vi "Project Save for Previous.vi"(7 "LabVIEW Previous Version":T1=enum."2015", 8 "Error In":errorcluster) -> (0 "Error Out":errorcluster, 3 "Destination":path)   [LabVIEW 2017, in "Scripts.lvlib"]
doc: "Saves a project to a previous version of LabVIEW. The output is saved to \"<project root>\\target\\<Target Version>\", where \"<project root>\" is the folder that contains the LabVIEW project file (.lvproj) and \"<Target Version>\" is the previous version of LabVIEW, such as \"15.0\" for LabVIEW 2015."
uses:
  Scripts.lvlib
  Controls/LabVIEW Versions.ctl
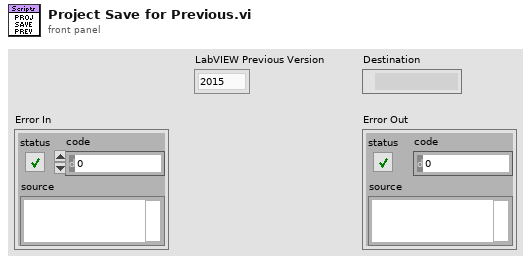
[diagram p1: front panel]
types:
  T1 = typedef "Scripts.lvlib/LabVIEW Versions.ctl" = enum16{"2009", "2010", "2011", "2012", "2013", "2014", "2015", "2016", "2017", "2018"}
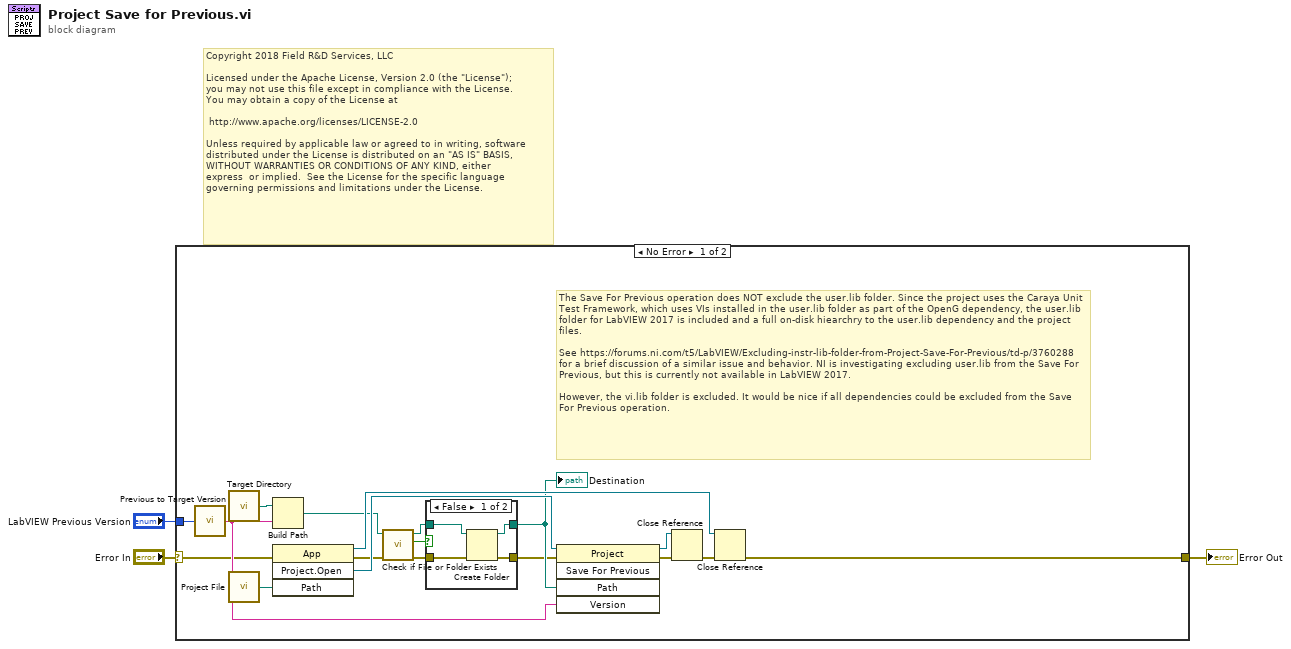
[diagram p0: block diagram]
diagram:
  # "Copyright 2018 Field R&D Services, LLC\n\nLicensed under the Apache License, Version 2.0 (the \"License\");\nyou may not use this file except in compliance with the License.\nYou may obtain a copy of the License at\n\n\thttp://www.apache.org/licenses/LICENSE-2.0\n\nUnless required by applicable law or agreed to in writing, software\ndistributed under the License is distributed on an \"AS IS\" BASIS,\nWITHOUT WARRANTIES OR CONDITIONS OF ANY KIND, either \nexpress  or implied.  See the License for the specific language \ngoverning permissions and limitations under the License."
  n1 = case shown="No Error" "Error In" {
    selector: "Error In" -> [w4 w28]
    tunnel: [w16 w28] -> w3
    tunnel: "LabVIEW Previous Version" -> [w9 _]
    frame No Error {
      # "The Save For Previous operation does NOT exclude the user.lib folder. Since the project uses the Caraya Unit Test Framework, which uses VIs installed in the user.lib folder as part of the OpenG dependency, the user.lib folder for LabVIEW 2017 is included and a full on-disk hiearchry to the user.lib dependency and the project files.\n\nSee https://forums.ni.com/t5/LabVIEW/Excluding-instr-lib-folder-from-Project-Save-For-Previous/td-p/3760288 for a brief discussion of a similar issue and behavior. NI is investigating excluding user.lib from the Save For Previous, but this is currently not available in LabVIEW 2017.\n\nHowever, the vi.lib folder is excluded. It would be nice if all dependencies could be excluded from the Save For Previous operation."
      n2 = call "Previous to Target Version.vi"("Previous Version"=w9) -> ("Target Version"=w7:string)
      n3 = call "Target Directory.vi"() -> ("Target Directory"=w5:path)
      n4 = call "Project File.vi"() -> ("Project File"=w6:path)
      n5 = Build Path(base path=w5, name or relative path=w7) -> (appended path=w8:path)
      n6 = invoke class="App" method="Project.Open"(error in=w4, "Path"=w6) -> (reference out=w18:refnum<vi>, error out=w15:errorcluster, "Project:Open"=w21:refnum<vi>)  [unwired: 2 in, 1 out]
      n7 = call <vilib>:"Check if File or Folder Exists.vi"("error in (no error)"=w15, "path"=w8) -> ("error out"=w11:errorcluster, "file or folder exists?"=w14:bool, "dup path"=w13:path)  [unwired: 7 in]
      n8 = case shown="False" w14 {
        tunnel: w13 -> [w25 w27]
        tunnel: [w22 w27] -> w12
        tunnel: w11 -> [w24 w26]
        tunnel: [w23 w26] -> w10
        frame False {
          n9 = Create Folder(path (use dialog)=w25, error in=w24) -> (created path=w22:path, error out=w23:errorcluster)  [unwired: 1 in, 1 out]
        }
        frame True {
        }
      }
      "Destination" <- w12
      n10 = invoke class="Project" method="Save For Previous"(reference=w21, error in=w10, "Path"=w12, "Version"=w7) -> (reference out=w19:refnum<vi>, error out=w20:errorcluster)  [unwired: 1 in, 3 out]
      n11 = Close Reference(reference=w19, error in (no error)=w20) -> (error out=w17:errorcluster)
      n12 = Close Reference(reference=w18, error in (no error)=w17) -> (error out=w16:errorcluster)
    }
    frame Error {
    }
  }
  "Error Out" <- w3
